vi "Set Signal Configuration.vi"(8 "error in":errorcluster, 10 "Selected Channels":T1 {"CRC"."Data Type" items=["Signed", "Unsigned", "IEEE Float"]; "Rolling Counter"."Data Type" items=["Signed", "Unsigned", "IEEE Float"]; "Input Channels"."Data Type" items=["Signed", "Unsigned", "IEEE Float"]}, 11 "Parent Ref":T4=18446744073709551615 format="%.0x") -> (0 "error out":errorcluster, 3 "Parent Ref Out":T4=18446744073709551615 format="%.0x")   [LabVIEW 2021, in "LIN Frame Protection Addon Shared.lvlib"]
uses:
  LIN Frame Protection Addon Shared.lvlib
  <vilib>/NI VeriStand/Custom Device API/Custom Device Item Ref.ctl
  Types/FrameConfiguration.ctl
  Types/InputChannelConfiguration.ctl
  Types/Protection Type.ctl
  GUID Lookup.vi
  <vilib>/NI VeriStand/Custom Device API/Set Item Property (Variant).vi
  <vilib>/NI VeriStand/Custom Device API/Custom Device API.lvlib
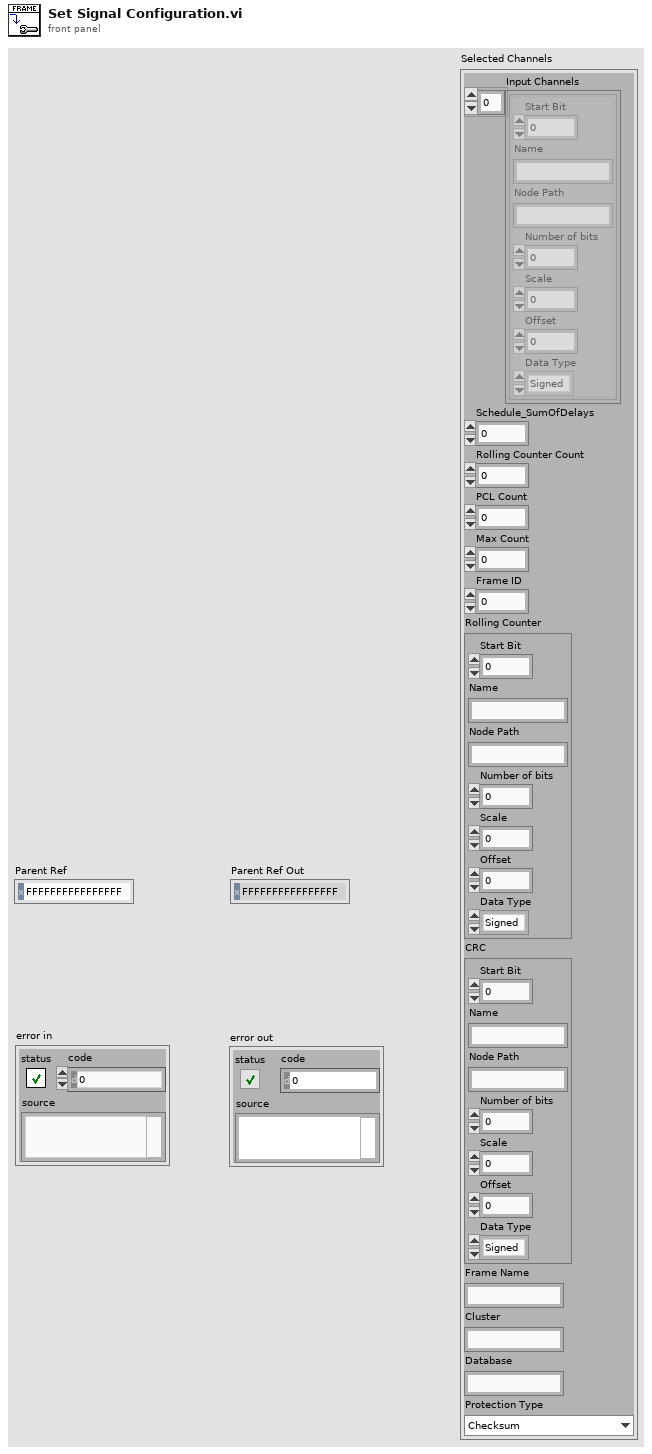
[diagram p1: front panel]
types:
  T1 = typedef "LIN Frame Protection Addon Shared.lvlib/FrameConfiguration.ctl" = cluster{"Input Channels":T2[], "Schedule_SumOfDelays":dbl, "Rolling Counter Count":dbl, "PCL Count":u64, "Max Count":dbl, "Frame ID":u32, "Rolling Counter":T2, "CRC":T2, "Frame Name":string, "Cluster":string, "Database":string, "Protection Type":T3}
  T2 = typedef "LIN Frame Protection Addon Shared.lvlib/InputChannelConfiguration.ctl" = cluster{"Start Bit":i32, "Name":string, "Node Path":string, "Number of bits":i32, "Scale":dbl, "Offset":dbl, "Data Type":u32}
  T3 = typedef "LIN Frame Protection Addon Shared.lvlib/Protection Type.ctl" = enum16{"Checksum", "CRC", "None (Counter Only)"}
  T4 = typedef "Custom Device API.lvlib/Custom Device Item Ref.ctl" = u64
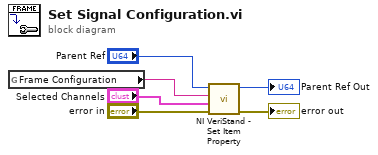
[diagram p0: block diagram]
diagram:
  n1 = global read "GUID Lookup.vi" "Frame Configuration"() -> (w2:string)
  n2 = call-poly <vilib>:"NI VeriStand - Set Item Property.vi"("error in (no error)"="error in", "Value"="Selected Channels", "Property Name"=w2, "Item Ref in"="Parent Ref") -> ("error out"=→"error out":errorcluster, "Item Ref out"=→"Parent Ref Out":T4)  [unwired: 5 in, 1 out]
